vi "DataSocketServer-receiver.vi"() -> ()   [LabVIEW 2020]
panel:
  out "Gauge":i32(knob) scale=0.0..100.0
  out "Numeric":i32
  out "Waveform Chart":i32(graph)
  in  "stop":bool
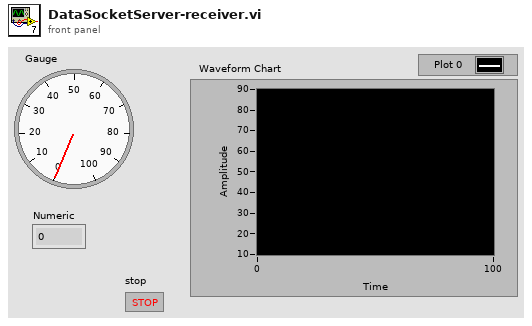
[diagram p1: front panel]
types:
  T1 = enum16{"Read", "Write", "ReadWrite", "BufferedRead", "BufferedReadWrite"}
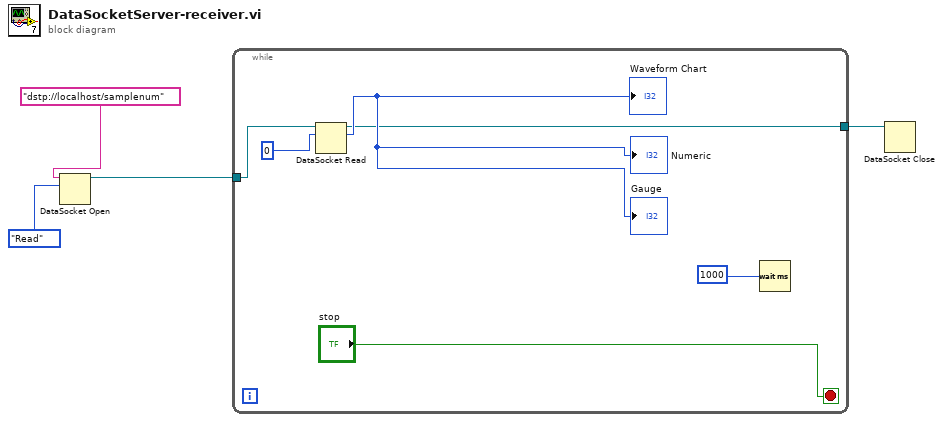
[diagram p0: block diagram]
diagram:
  n1 = DataSocket Open(10:T1."Read" ("mode"), 11:"dstp://localhost/samplenum") -> (3:w3:refnum<k13>)  [unwired: 2 in, 1 out]
  n2 = while {
    tunnel: w3 -> [w8]
    tunnel: [w6] -> w1
    stop <- "stop" stop-if-true
    n3 = DataSocket Read(10:0, 11:w8) -> (2:→"Waveform Chart" →"Numeric" →"Gauge":i32, 3:w6:refnum<k13>)  [unwired: 3 in, 5 out]
    n4 = Wait (ms)(milliseconds to wait=1000) -> ()  [unwired: 1 out]
  }
  n5 = DataSocket Close(11:w1) -> ()  [unwired: 2 in, 2 out]
